vi "fFIFO Throughput.vi"(0 "Elements in FIFO":u32(graph), 10 "Loop Time":u32, 11 "Array":i16[](array[numeric])) -> (1 "FIFO Overflow":bool, 2 "Inst. Throughput":dbl format="%#_6p", 3 "Average Throughput":dbl(graph))   [LabVIEW 2014]
uses:
  <vilib>/ptbypt/NI_PtbyPt.lvlib
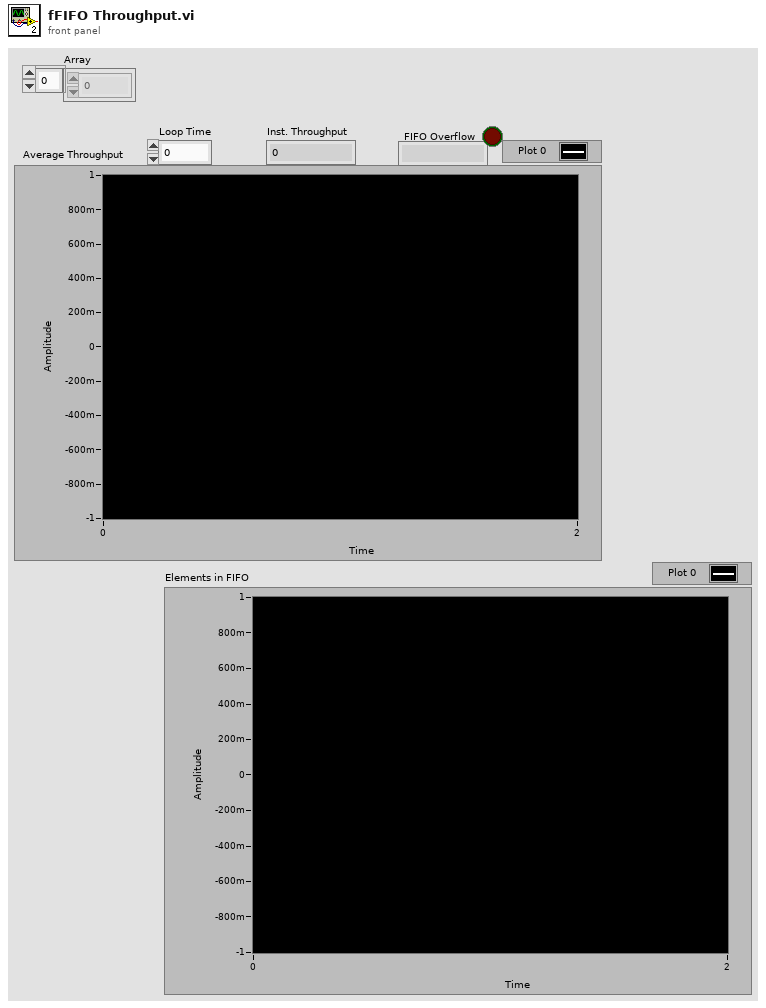
[diagram p1: front panel]
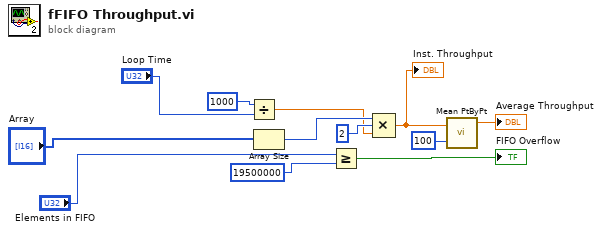
[diagram p0: block diagram]
diagram:
  n1 = Divide(x=u32 1000, y="Loop Time") -> (x/y=w9:dbl)
  n2 = Array Size(array="Array") -> (size(s)=w12:i32)
  n3 = Greater Or Equal?(x="Elements in FIFO", y=u32 19500000) -> (x >= y?=→"FIFO Overflow":bool)
  n4 = Compound Arithmetic op=MULTIPLY(w12, 2 ("y"), w9) -> (w7:dbl)
  "Inst. Throughput" <- w7
  n5 = call <vilib>:"Mean PtByPt.vi"("x"=w7, "sample length"=100) -> ("mean"=→"Average Throughput":dbl)  [unwired: 2 in, 1 out]
